vi "6_SumorProduct1toN.vi"() -> ()   [LabVIEW 2015]
panel:
  in  "Product or Sum?":bool=TRUE
  out "Sum of 1 to N for multiples of 3 & 5":u32
  in  "Enter a number":u32
  # "Product"
  # "Sum"
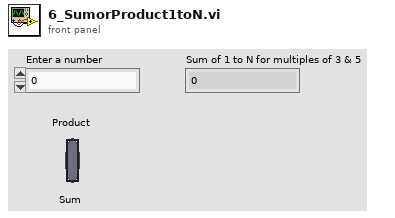
[diagram p1: front panel]
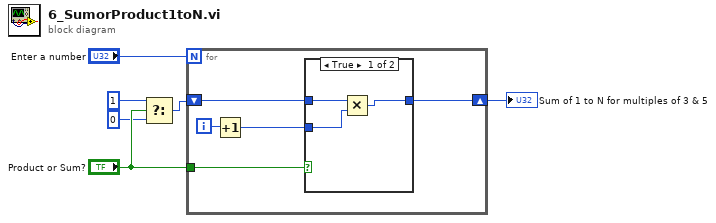
[diagram p0: block diagram]
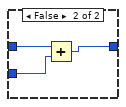
[diagram p2: hidden frame]
diagram:
  n1 = Select(t=1, s="Product or Sum?", f=0) -> (s? t:f=w3:i32)
  n2 = for {
    N: "Enter a number" -> [_]
    shift-right: [w9] -> w4
    shift-left: w3 -> [w10]
    tunnel: "Product or Sum?" -> [w7]
    i -> [w11]
    n3 = Increment(x=w11) -> (x+1=w8:i32)
    n4 = case shown="True" w7 {
      tunnel: w10 -> [w14 w17]
      tunnel: [w13 w16] -> w9
      tunnel: w8 -> [w12 w15]
      frame True {
        n5 = Multiply(x=w14, y=w12) -> (x*y=w13:i32)
      }
      frame False {
        n6 = Add(x=w17, y=w15) -> (x+y=w16:i32)
      }
    }
  }
  "Sum of 1 to N for multiples of 3 & 5" <- w4
